vi "VCS Get Protocol Stack Name.vi"(8 "error in (no error)":errorcluster, 11 "axis in":cluster{"keyHandle":u32, "nodeId":u16}={"keyHandle"=0, "nodeId"=1}) -> (0 "error out":errorcluster, 2 "protocolStackName":string, 3 "axis out":cluster{"keyHandle":u32, "nodeId":u16}={"keyHandle"=0, "nodeId"=1})   [LabVIEW 2019, in "maxonEPOS.lvlib"]
doc: "<B>VCS Get Protocol Stack Name</B> returns the protocol stack name to corresponding handle."
uses:
  Examples/maxonEPOS.lvlib
  Resources/EposCmd.dll
  Resources/EposCmd64.dll
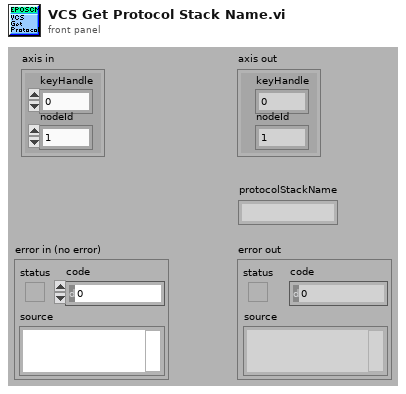
[diagram p1: front panel]
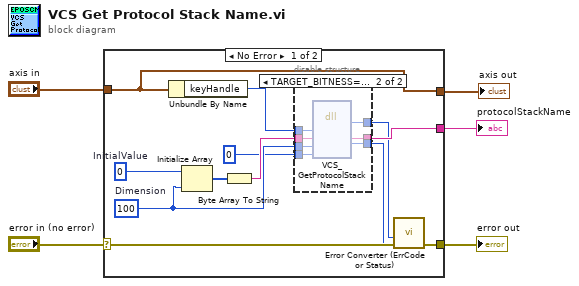
[diagram p0: block diagram]
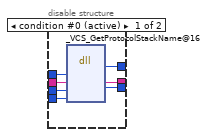
[diagram p2: hidden frame]
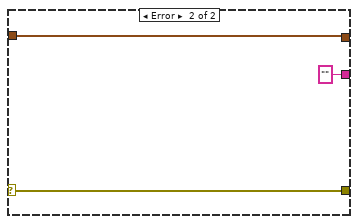
[diagram p3: hidden frame]
diagram:
  n1 = case shown="No Error" "error in (no error)" {
    selector: "error in (no error)" -> [w16 w34]
    tunnel: [w15 w34] -> w4
    tunnel: [w17 "" ("pProtocolStackName")] -> w3
    tunnel: "axis in" -> [w7 w33]
    tunnel: [w7 w33] -> w1
    frame No Error {
      w11 = u8 0  # InitialValue
      w9 = 100  # Dimension
      n2 = Unbundle By Name(w7) -> ("keyHandle"=w13:u32)
      n3 = Initialize Array(w11, w9) -> (w12:u8[])
      n4 = Byte Array To String(unsigned byte array=w12) -> (string=w10:string)
      n5 = disable-structure shown="TARGET_BITNESS==64" {
        disable-tunnel: [w24 w31] -> w17
        disable-tunnel: [w23 w30] -> w14
        disable-tunnel: w13 -> [w22 w29]
        disable-tunnel: w10 -> [w21 w28]
        disable-tunnel: w9 -> [w20 w27]
        disable-tunnel: u32 0 ("pErrorCode") -> [w19 w26]
        disable-tunnel: [w18 w25] -> w6
        frame condition #0 (active) {
          n6 = dll-call lib="C:/workspace/project/scancon/sw/SSI_Tool/InstrumentsInterfaces/Motordriver/maxon EPOS/Resources/EposCmd.*" fn="_VCS_GetProtocolStackName@16"("KeyHandle"=w22, "pProtocolStackName"=w21, "MaxStrSize"=w20, "pErrorCode"=w19) -> (w18:i32, "pProtocolStackName"=w24:string, "pErrorCode"=w23:u32)  [unwired: 5 in, 2 out]
        }
        frame condition #1 {
          n7 = dll-call lib="C:/setup/Resources/EposCmd64.dll" fn="VCS_GetProtocolStackName" ("EposCmd.dll:_VCS_GetProtocolStackName@16")("KeyHandle"=w29, "pProtocolStackName"=w28, "MaxStrSize"=w27, "pErrorCode"=w26) -> ("Rückgabetyp"=w25:i32, "pProtocolStackName"=w31:string, "pErrorCode"=w30:u32)  [unwired: 5 in, 2 out]
        }
      }
      n8 = call "Error Converter (ErrCode or Status).vi"("error code"=w14, "return type"=w6, "error in (no error)"=w16) -> ("error out"=w15:errorcluster)  [unwired: 7 in]
    }
    frame Error {
    }
  }
  "protocolStackName" <- w3
  "error out" <- w4
  "axis out" <- w1
